vi "task_process_read-image_name.vi"(8 "error in (no error)":errorcluster, 11 "image_name":string) -> (0 "error out":errorcluster, 3 "pid []":i32[](array[numeric]))   [LabVIEW 2015, in "em-lv-cmd-utilities.lvlib"]
uses:
  em-lv-cmd-utilities.lvlib
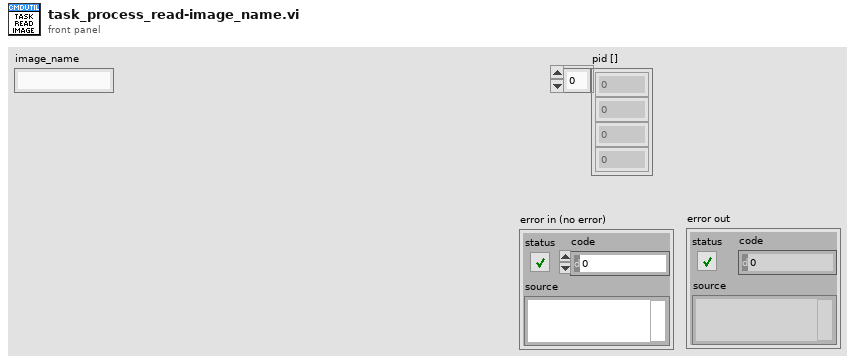
[diagram p1: front panel]
types:
  T1 = cluster{"image_name []":string[], "pid []":i32[], "session_name []":string[], "session_number []":i32[], "memory_usage []":dbl[]}
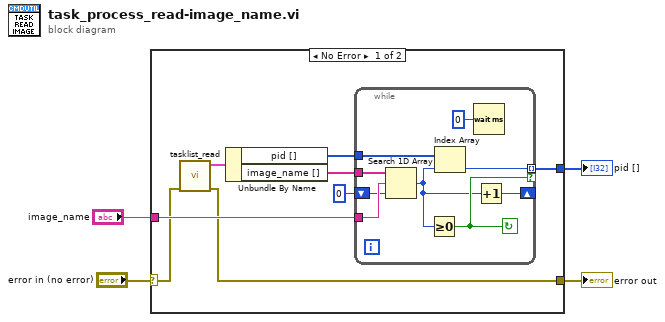
[diagram p0: block diagram]
diagram:
  n1 = case shown="No Error" "error in (no error)" {
    selector: "error in (no error)" -> [w6 w22]
    tunnel: "image_name" -> [w12 _]
    tunnel: [w7 _] -> w3
    tunnel: [w5 w22] -> w1
    frame No Error {
      n2 = call "tasklist_read.vi"("error in (no error)"=w6) -> ("error out"=w5:errorcluster, "tasklist"=w11:T1)  [unwired: 9 in]
      n3 = Unbundle By Name(w11) -> ("pid []"=w9:i32[], "image_name []"=w10:string[])
      n4 = while {
        tunnel: w12 -> [w20]
        tunnel: w10 -> [w21]
        tunnel: w9 -> [w18]
        tunnel: [w19] -> w7 mode=indexing if=w17
        shift-right: [w14] -> _
        shift-left: 0 ("index of element") -> [w15]
        stop <- w17 continue-if-true
        n5 = Search 1D Array(1D array=w21, element=w20, start index (0)=w15) -> (index of element=w16:i32)
        n6 = Greater Or Equal To 0?(x=w16) -> (x >= 0?=w17:bool)
        n7 = Index Array(array=w18, index=w16) -> (element=w19:i32)
        n8 = Wait (ms)(milliseconds to wait=u32 0) -> ()  [unwired: 1 out]
        n9 = Increment(x=w16) -> (x+1=w14:i32)
      }
    }
    frame Error {
    }
  }
  "pid []" <- w3
  "error out" <- w1
